vi "Read motorData.vi"(8 "error in (no error)":errorcluster, 11 "MotorController in":refnum<class "MotorController.lvclass">) -> (0 "error out":errorcluster, 2 "motorData":T1={"Velo (RPM)"=0, "MotorTemp(C)"=0, "CtrlTemp(C)"=0, "DcLinkVolt(V)"=0.0, "ErrorCode"=0.0, "isAlive"=FALSE, "motorControllerState"=1, "motorStatus"={"isReady"=FALSE, "isOn"=FALSE, "isOperEn"=FALSE, "isFault"=FALSE, "isVoltEn"=FALSE, "targetReached"=FALSE, "isWarning"=FALSE}} {"motorControllerState" items=["unknown"=1, "boot-up"=0, "stopped"=4, "operational"=5, "pre-operational"=127, "connection lost"=128]}, 3 "MotorController out":refnum<class "MotorController.lvclass">)   [LabVIEW 2017, in "MotorController.lvclass"]
uses:
  MotorController.lvclass
  MotorData.ctl
  MotorStatus.ctl
  MotorController.lvclass/MotorController.ctl
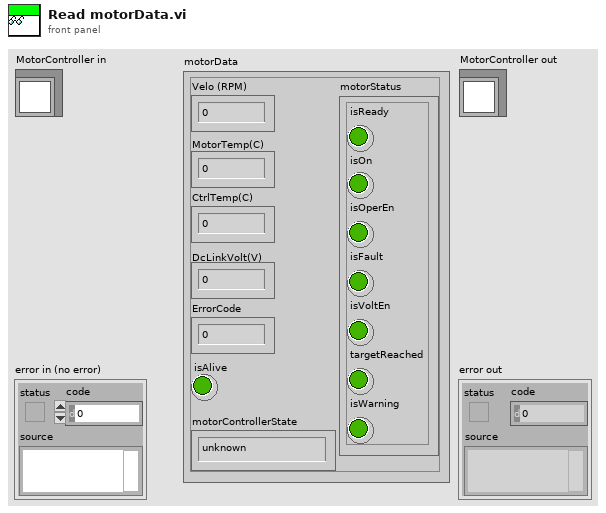
[diagram p1: front panel]
types:
  T1 = typedef "MotorData.ctl" = cluster{"Velo (RPM)":i32, "MotorTemp(C)":u8, "CtrlTemp(C)":u8, "DcLinkVolt(V)":dbl, "ErrorCode":dbl, "isAlive":bool, "motorControllerState":u16, "motorStatus":T2}
  T2 = typedef "MotorStatus.ctl" = cluster{"isReady":bool, "isOn":bool, "isOperEn":bool, "isFault":bool, "isVoltEn":bool, "targetReached":bool, "isWarning":bool}
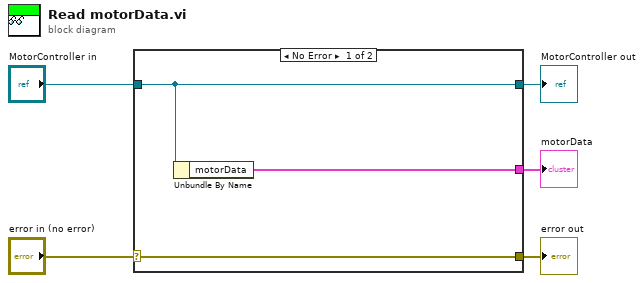
[diagram p0: block diagram]
diagram:
  n1 = case shown="No Error" "error in (no error)" {
    selector: "error in (no error)" -> [w8 w9]
    tunnel: [w8 w9] -> w4
    tunnel: [w7 w10] -> w2
    tunnel: "MotorController in" -> [w7 w10]
    tunnel: [w6 _] -> w1
    frame No Error {
      n2 = Unbundle By Name(w7) -> ("motorData"=w6:T1)
    }
    frame Error {
    }
  }
  "error out" <- w4
  "MotorController out" <- w2
  "motorData" <- w1
